vi "GV galvo scan direction.vi"() -> ()   [LabVIEW 2017]
panel:
  out "Galvo_scan_direction":bool
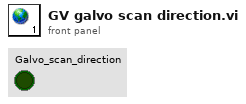
[diagram p1: front panel]
diagram:
